vi "Add Object.vi"(11 "Core Data in":T1) -> (3 "Core Data out":T1)   [LabVIEW 2020, in "Amnesia.lvlib"]
uses:
  Amnesia.lvlib
  Scene/Scene.lvclass
  Core Data.ctl
  Scene/Mouse Button Held.ctl
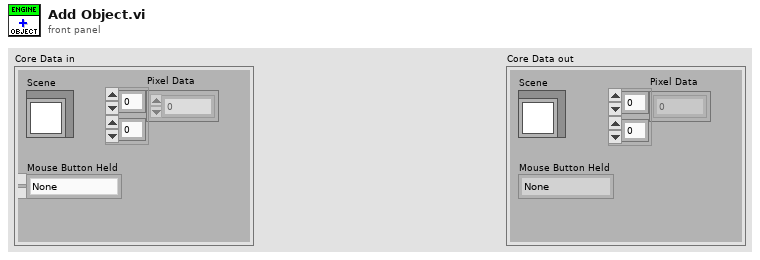
[diagram p1: front panel]
types:
  T1 = typedef "Amnesia.lvlib/Core Data.ctl" = cluster{"Pixel Data":u32[][], "Scene":refnum<class "Scene.lvclass">, "Mouse Button Held":T2}
  T2 = typedef "Scene.lvclass/Mouse Button Held.ctl" = enum16{"None", "Left", "Middle", "Right"}
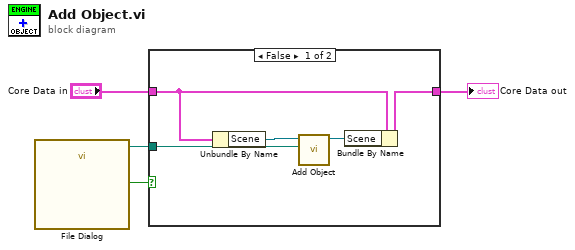
[diagram p0: block diagram]
diagram:
  n1 = call "File Dialog"() -> ("selected path"=w1:path, "cancelled"=w2:bool)  [unwired: 12 in, 2 out]
  n2 = case shown="False" w2 {
    tunnel: "Core Data in" -> [w8 w10]
    tunnel: [w6 w10] -> w3
    tunnel: w1 -> [w5 _]
    frame False {
      n3 = Unbundle By Name(w8) -> ("Scene"=w9:refnum<class "Scene.lvclass">)
      n4 = call "Add Object.vi"("OBJ File"=w5, "Scene in"=w9) -> ("Scene out"=w7:refnum<class "Scene.lvclass">)  [unwired: 8 in, 1 out]
      n5 = Bundle By Name(cluster=w8, "Scene"=w7) -> (w6:T1)
    }
    frame True {
    }
  }
  "Core Data out" <- w3
